vi "Config_Convert Falcon Cluster to Motion Magic Cluster.vi"(11 "Talon FX Configurables":T1 {"diff1Term" items=["Integrated Sensor"=1, "Sensor Sum (S0 + S1)"=9, "Sensor Difference (D0 - D1)"=10, "Remote Source 0"=11, "Remote Source 1"=12, "None"=14, "Software Emulated"=15]; "diff0Term" items=["Integrated Sensor"=1, "Sensor Sum (S0 + S1)"=9, "Sensor Difference (D0 - D1)"=10, "Remote Source 0"=11, "Remote Source 1"=12, "None"=14, "Software Emulated"=15]; "sum1Term" items=["Integrated Sensor"=1, "Sensor Sum (S0 + S1)"=9, "Sensor Difference (D0 - D1)"=10, "Remote Source 0"=11, "Remote Source 1"=12, "None"=14, "Software Emulated"=15]; "sum0Term" items=["Integrated Sensor"=1, "Sensor Sum (S0 + S1)"=9, "Sensor Difference (D0 - D1)"=10, "Remote Source 0"=11, "Remote Source 1"=12, "None"=14, "Software Emulated"=15]; "auxiliaryPID"."selectedFeedbackSensor" items=["Integrated Sensor"=1, "Sensor Sum (S0 + S1)"=9, "Sensor Difference (D0 - D1)"=10, "Remote Source 0"=11, "Remote Source 1"=12, "None"=14, "Software Emulated"=15]; "primaryPID"."selectedFeedbackSensor" items=["Integrated Sensor"=1, "Sensor Sum (S0 + S1)"=9, "Sensor Difference (D0 - D1)"=10, "Remote Source 0"=11, "Remote Source 1"=12, "None"=14, "Software Emulated"=15]; "Base Configurables"."velocityMeasurementPeriod" items=["Period_1ms"=1, "Period_2ms"=2, "Period_5ms"=5, "Period_10ms"=10, "Period_20ms"=20, "Period_25ms"=25, "Period_50ms"=50, "Period_100ms"=100]}) -> (3 "MM":T16)   [LabVIEW 2020]
uses:
  TypeDefs/Cluster_Motion Magic Parameters.ctl
  <vilib>/Rock Robotics/WPI/ThirdParty/Phoenix-LabVIEW/Motor Controller/Controls/CTRE_Phoenix_MotorControl_VelocityMeasurementPeriod.ctl
  <vilib>/Rock Robotics/WPI/ThirdParty/Phoenix-LabVIEW/Motor Controller/Controls/CTRE_Phoenix_MotorControl_SlotStructure.ctl
  <vilib>/Rock Robotics/WPI/ThirdParty/Phoenix-LabVIEW/Motor Controller/Controls/CTRE_Phoenix_MotorControl_RemoteSourceType.ctl
  <vilib>/Rock Robotics/WPI/ThirdParty/Phoenix-LabVIEW/Motor Controller/Controls/CTRE_Phoenix_MotorControl_FilterStruct.ctl
  <vilib>/Rock Robotics/WPI/ThirdParty/Phoenix-LabVIEW/Controls/CTRE_Phoenix_CustomParamConfiguration.ctl
  <vilib>/Rock Robotics/WPI/ThirdParty/Phoenix-LabVIEW/Motor Controller/Controls/CTRE_Phoenix_MotorControl_BaseConfigurables.ctl
  <vilib>/Rock Robotics/WPI/ThirdParty/Phoenix-LabVIEW/Motor Controller/Controls/CTRE_Phoenix_MotorControl_FeedbackDevice_TalonFX.ctl
  <vilib>/Rock Robotics/WPI/ThirdParty/Phoenix-LabVIEW/Motor Controller/Controls/CTRE_Phoenix_MotorControl_LimitSwitchSource_Local.ctl
  <vilib>/Rock Robotics/WPI/ThirdParty/Phoenix-LabVIEW/Motor Controller/Controls/CTRE_Phoenix_MotorControl_LimitSwitchNormal.ctl
  <vilib>/Rock Robotics/WPI/ThirdParty/Phoenix-LabVIEW/Motor Controller/Controls/CTRE_Phoenix_MotorControl_SupplyCurrentLimitConfiguration.ctl
  <vilib>/Rock Robotics/WPI/ThirdParty/Phoenix-LabVIEW/Motor Controller/Controls/CTRE_Phoenix_MotorControl_StatorCurrentLimitConfiguration.ctl
  <vilib>/Rock Robotics/WPI/ThirdParty/Phoenix-LabVIEW/Motor Controller/Controls/CTRE_Phoenix_MotorControl_MotorCommutation_TalonFX.ctl
  <vilib>/Rock Robotics/WPI/ThirdParty/Phoenix-LabVIEW/CANCoder/Controls/CTRE_Phoenix_CANcoder_AbsoluteSensorRange.ctl
  <vilib>/Rock Robotics/WPI/ThirdParty/Phoenix-LabVIEW/CANCoder/Controls/CTRE_Phoenix_CANcoder_SensorInitializationStrategy.ctl
  <vilib>/Rock Robotics/WPI/ThirdParty/Phoenix-LabVIEW/Motor Controller/Controls/CTRE_Phoenix_MotorControl_TalonFXMotorControllerConfigurables.ctl
panel:
  # "Sum and Diff terms are ways to select more than one sensor as a feedback device. \n Sum 0 is the first feedback device to be used for the Sum term.\n Sum 1 is the feedback device to be added to Sum 0 for the Sum term.\n Diff 0 and Diff 1 work in a similar manner."
  # "These are only applicable\nif using a remote limit switch.\n\nLocal limit switches/no limit\nswitches do not use this."
  # "Current is below Current Limit AND\n\n(Requested output is weaker** than applied motor\noutput OR is in the opposite direction).\n/\nMotor output is set to requested output."
  # "Current is above Threshold Current for Threshold Time\n/\nReduce motor output (towards neutral)."
  # "Current is below Current Limit.\n/\nRamp motor output towards requested output."
  # "Current is above Current Limit.\n/\nReduce motor output (towards neutral)."
  # "*If the configured Peak Threshold is less than the Continuous Threshold, the applied Peak Threshold is set equal to the Configured Continuous Threshold in firmware.\n** Both requested output and applied motor output are in the same direction, and requested output is closer to neutral."
  # "False: Primary Output = PID[0] + PID[1]  ---  Auxiliary Output = PID[0] - PID[1]\nTrue:  Primary Output = PID[0] - PID[1] --- Auxiliary Output = PID[0] + PID[1]"
  # "Enable the motion profile executor to perform linear interpolation between profile points.  Defaults to True."
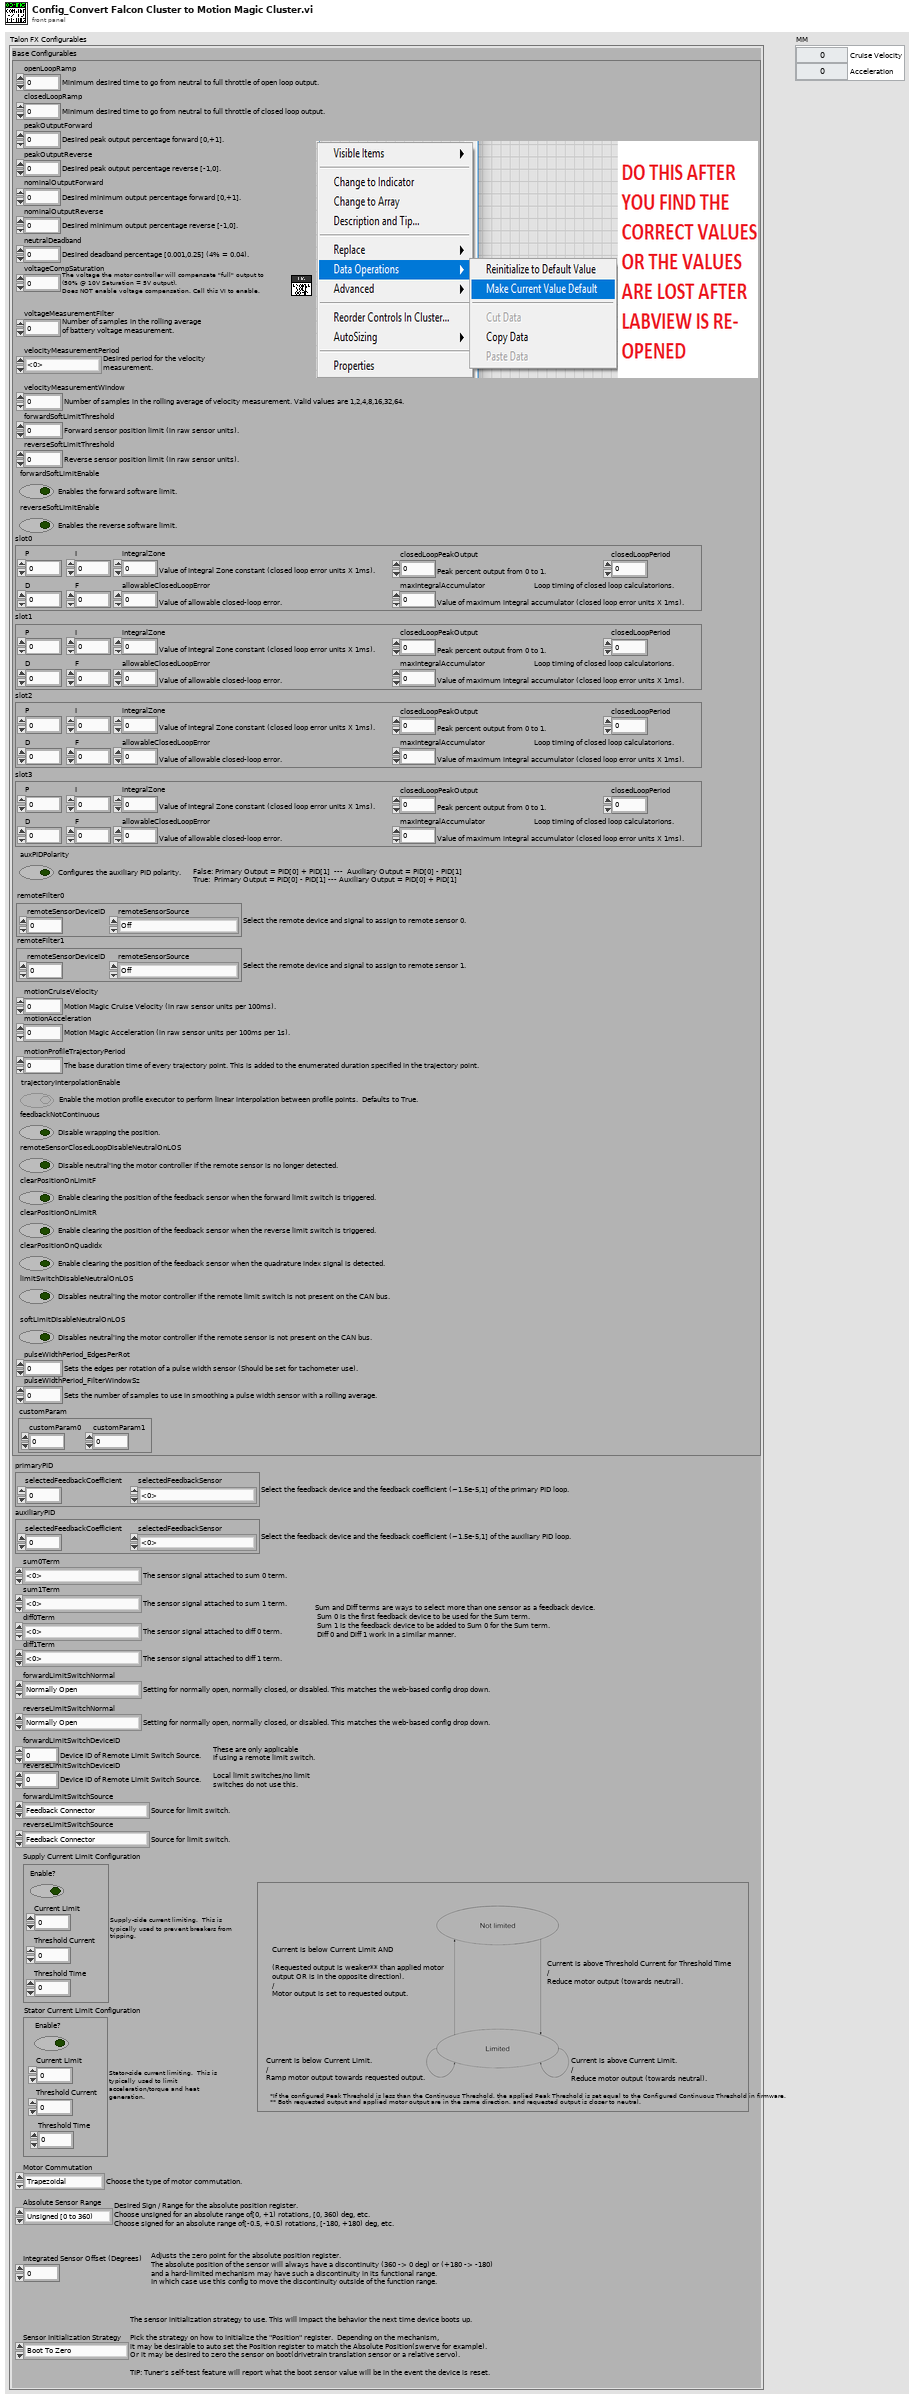
[diagram p1: front panel]
types:
  T1 = typedef "CTRE_Phoenix_MotorControl_TalonFXMotorControllerConfigurables.ctl" = cluster{"Base Configurables":T2, "primaryPID":cluster{"selectedFeedbackCoefficient":dbl, "selectedFeedbackSensor":T8}, "auxiliaryPID":cluster{"selectedFeedbackCoefficient":dbl, "selectedFeedbackSensor":T8}, "forwardLimitSwitchNormal":T9, "reverseLimitSwitchNormal":T9, "forwardLimitSwitchDeviceID":i32, "reverseLimitSwitchDeviceID":i32, "forwardLimitSwitchSource":T10, "reverseLimitSwitchSource":T10, "sum0Term":T8, "sum1Term":T8, "diff0Term":T8, "diff1Term":T8, "Supply Current Limit Configuration":T11, "Stator Current Limit Configuration":T12, "Motor Commutation":T13, "Absolute Sensor Range":T14, "Integrated Sensor Offset (Degrees)":dbl, "Sensor Initialization Strategy":T15}
  T2 = typedef "CTRE_Phoenix_MotorControl_BaseConfigurables.ctl" = cluster{"openLoopRamp":dbl, "closedLoopRamp":dbl, "peakOutputForward":dbl, "peakOutputReverse":dbl, "nominalOutputForward":dbl, "nominalOutputReverse":dbl, "neutralDeadband":dbl, "voltageCompSaturation":dbl, "voltageMeasurementFilter":i32, "velocityMeasurementPeriod":T3, "velocityMeasurementWindow":i32, "forwardSoftLimitThreshold":i32, "reverseSoftLimitThreshold":i32, "forwardSoftLimitEnable":bool, "reverseSoftLimitEnable":bool, "slot0":T4, "slot1":T4, "slot2":T4, "slot3":T4, "auxPIDPolarity":bool, "remoteFilter0":T5, "remoteFilter1":T5, "motionCruiseVelocity":i32, "motionAcceleration":i32, "motionProfileTrajectoryPeriod":i32, "feedbackNotContinuous":bool, "remoteSensorClosedLoopDisableNeutralOnLOS":bool, "clearPositionOnLimitF":bool, "clearPositionOnLimitR":bool, "clearPositionOnQuadIdx":bool, "limitSwitchDisableNeutralOnLOS":bool, "softLimitDisableNeutralOnLOS":bool, "pulseWidthPeriod_EdgesPerRot":i32, "pulseWidthPeriod_FilterWindowSz":i32, "customParam":T7, "trajectoryInterpolationEnable":bool}
  T3 = typedef "CTRE_Phoenix_MotorControl_VelocityMeasurementPeriod.ctl" = u16
  T4 = typedef "CTRE_Phoenix_MotorControl_SlotStructure.ctl" = cluster{"P":dbl, "I":dbl, "D":dbl, "F":dbl, "integralZone":dbl, "allowableClosedLoopError":i32, "maxIntegralAccumulator":dbl, "closedLoopPeakOutput":dbl, "closedLoopPeriod":i32}
  T5 = typedef "CTRE_Phoenix_MotorControl_FilterStruct.ctl" = cluster{"remoteSensorDeviceID":u8, "remoteSensorSource":T6}
  T6 = typedef "CTRE_Phoenix_MotorControl_RemoteSourceType.ctl" = enum16{"Off", "Talon SRX Selected Sensor", "Pigeon IMU Yaw", "Pigeon IMU Pitch", "Pigeon IMU Roll", "CANifier Quadrature", "CANifier PWM Input 0", "CANifier PWM Input 1", "CANifier PWM Input 2", "CANifier PWM Input 3", "Gadgeteer Pigeon Yaw", "Gadgeteer Pigeon Pitch", "Gadgeteer Pigeon Roll", "CANCoder"}
  T7 = typedef "CTRE_Phoenix_CustomParamConfiguration.ctl" = cluster{"customParam0":i32, "customParam1":i32}
  T8 = typedef "CTRE_Phoenix_MotorControl_FeedbackDevice_TalonFX.ctl" = i8
  T9 = typedef "CTRE_Phoenix_MotorControl_LimitSwitchNormal.ctl" = enum16{"Normally Open", "Normally Closed", "Disabled"}
  T10 = typedef "CTRE_Phoenix_MotorControl_LimitSwitchSource_Local.ctl" = enum16{"Feedback Connector", "Remote Talon SRX", "Remote CANifier", "Deactivated"}
  T11 = typedef "CTRE_Phoenix_MotorControl_SupplyCurrentLimitConfiguration.ctl" = cluster{"Enable?":bool, "Current Limit":dbl, "Threshold Current":dbl, "Threshold Time":dbl}
  T12 = typedef "CTRE_Phoenix_MotorControl_StatorCurrentLimitConfiguration.ctl" = cluster{"Enable?":bool, "Current Limit":dbl, "Threshold Current":dbl, "Threshold Time":dbl}
  T13 = typedef "CTRE_Phoenix_MotorControl_MotorCommutation_TalonFX.ctl" = enum16{"Trapezoidal"}
  T14 = typedef "CTRE_Phoenix_CANcoder_AbsoluteSensorRange.ctl" = enum16{"Unsigned [0 to 360)", "Signed [-180 to +180)"}
  T15 = typedef "CTRE_Phoenix_CANcoder_SensorInitializationStrategy.ctl" = enum16{"Boot To Zero", "Boot To Absolute Position"}
  T16 = typedef "Cluster_Motion Magic Parameters.ctl" = cluster{"Cruise Velocity":i32, "Acceleration":i32}
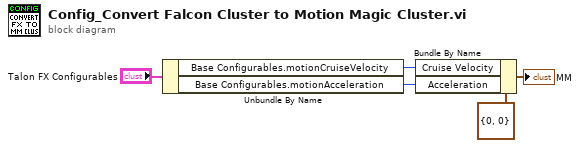
[diagram p0: block diagram]
diagram:
  n1 = Unbundle By Name("Talon FX Configurables") -> ("Base Configurables.motionCruiseVelocity"=w2:i32, "Base Configurables.motionAcceleration"=w1:i32)
  n2 = Bundle By Name(cluster=T16 {"Cruise Velocity"=0, "Acceleration"=0} ("MM"), "Cruise Velocity"=w2, "Acceleration"=w1) -> (→"MM":T16)
